vi "string_number_to_array.vi"(8 "string number":string, 11 "numeric length":i32) -> (3 "array number":u16[](array[numeric]))   [LabVIEW 2025]
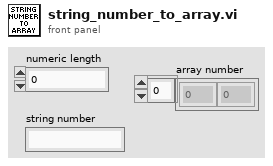
[diagram p1: front panel]
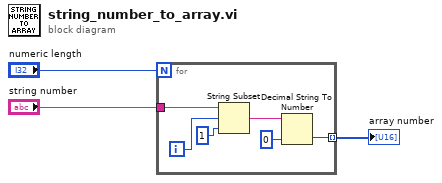
[diagram p0: block diagram]
diagram:
  n1 = for {
    N: "numeric length" -> [_]
    tunnel: "string number" -> [w9]
    tunnel: [w4] -> w1 mode=indexing
    i -> [w7]
    n2 = String Subset(string=w9, offset (0)=w7, length (rest)=1 ("length (rest)")) -> (substring=w6:string)
    n3 = Decimal String To Number(string=w6, default (0L)=u16 0 ("default (0 I32)")) -> (number=w4:u16)  [unwired: 1 in, 1 out]
  }
  "array number" <- w1
